vi "Tag Data.vi"(8 "error in (no error)":errorcluster, 11 "IFD_Tag in":refnum<class "IFD_Tag.lvclass">) -> (0 "error out":errorcluster, 2 "Data(Varient)":variant, 3 "IFD_Tag out":refnum<class "IFD_Tag.lvclass">)   [LabVIEW 2016, in "IFD_Tag.lvclass"]
uses:
  IFD_Tag.lvclass
  IFD_Tag.lvclass/IFD_Tag.ctl
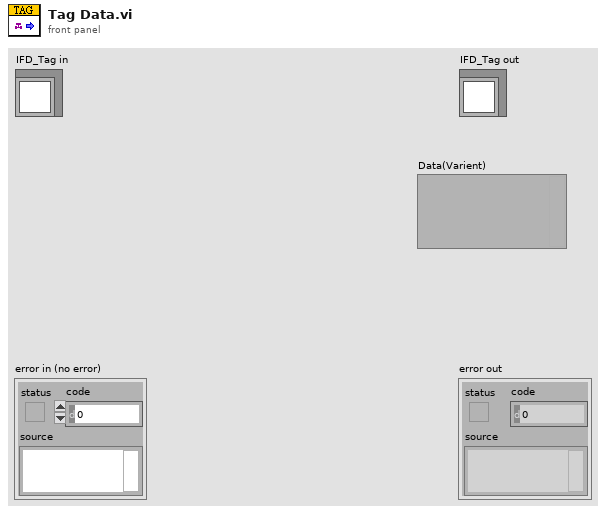
[diagram p1: front panel]
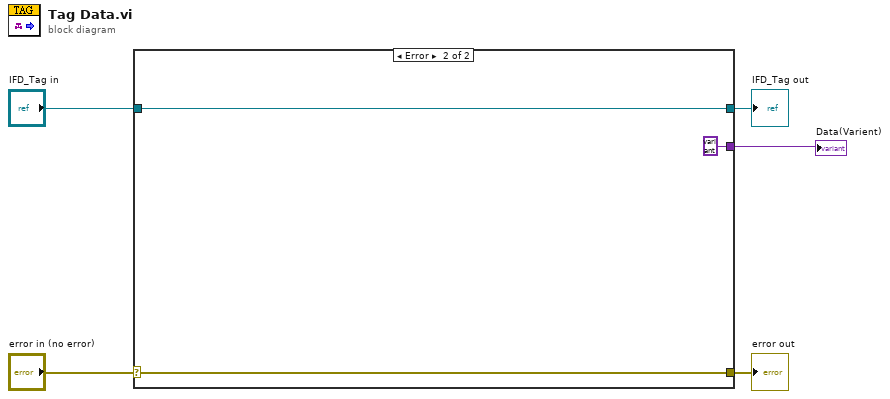
[diagram p0: block diagram]
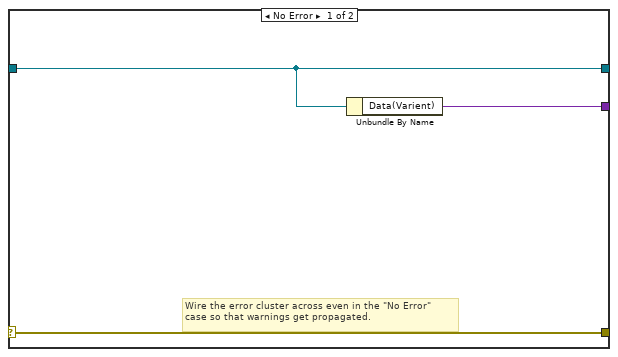
[diagram p2: hidden frame]
diagram:
  n1 = case shown="Error" "error in (no error)" {
    selector: "error in (no error)" -> [w8 w11]
    tunnel: [w8 w11] -> w4
    tunnel: [w7 w10] -> w2
    tunnel: "IFD_Tag in" -> [w7 w10]
    tunnel: [w6 variant ("Data(Varient)")] -> w1
    frame No Error {
      # "Wire the error cluster across even in the \"No Error\"\ncase so that warnings get propagated."
      n2 = Unbundle By Name(w7) -> ("Data(Varient)"=w6:variant)
    }
    frame Error {
    }
  }
  "error out" <- w4
  "IFD_Tag out" <- w2
  "Data(Varient)" <- w1
